vi "UI_Chose_Function.vi"() -> ()   [LabVIEW 2014]
panel:
  in  "报警门限及工作条件修改":bool
  in  "载荷谱修改":bool
  in  "齿轮箱独立调试":T1
  in  "陪试单元独立调试":T2
  in  "加载单元独立调试":T3
  in  "试验单元独立调试":T4
  in  "退出登录":T5
  in  "用户管理":T6
  in  "历史信息":T7
  in  "开始试验":T8
  # "轴承测试系统"
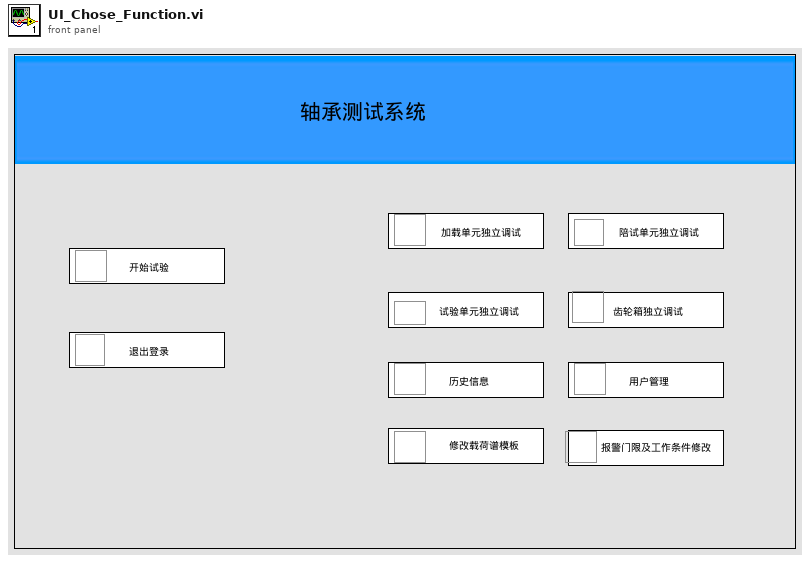
[diagram p1: front panel]
types:
  T1 = typedef "齿轮箱独立测试.ctl" = bool
  T2 = typedef "陪试单元独立调试.ctl" = bool
  T3 = typedef "加载单元独立调试.ctl" = bool
  T4 = typedef "试验单元独立调试.ctl" = bool
  T5 = typedef "退出登录1.ctl" = bool
  T6 = typedef "用户管理.ctl" = bool
  T7 = typedef "历史信息.ctl" = bool
  T8 = typedef "开始试验.ctl" = bool
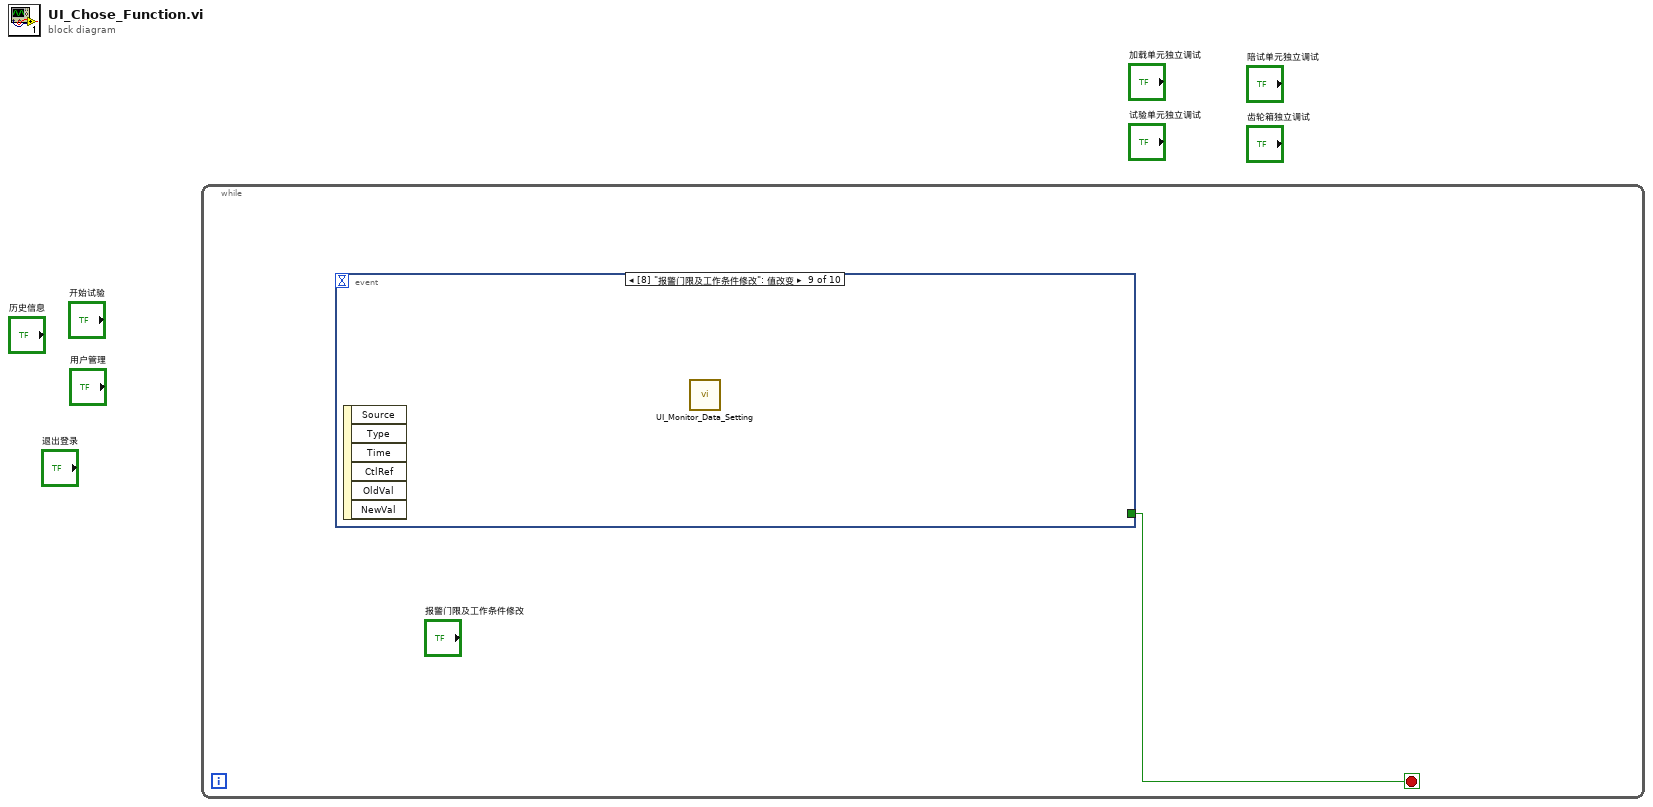
[diagram p0: block diagram]
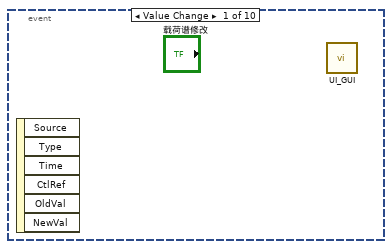
[diagram p2: hidden frame]
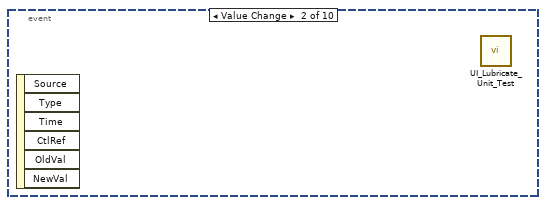
[diagram p3: hidden frame]
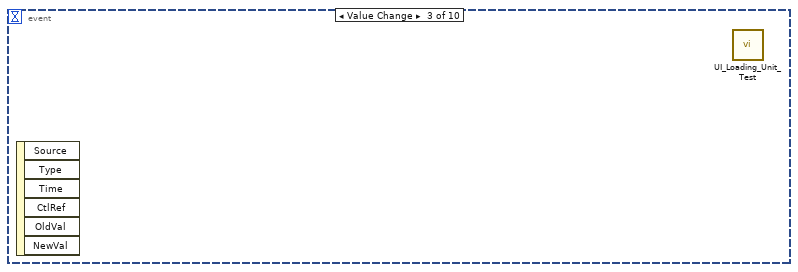
[diagram p4: hidden frame]
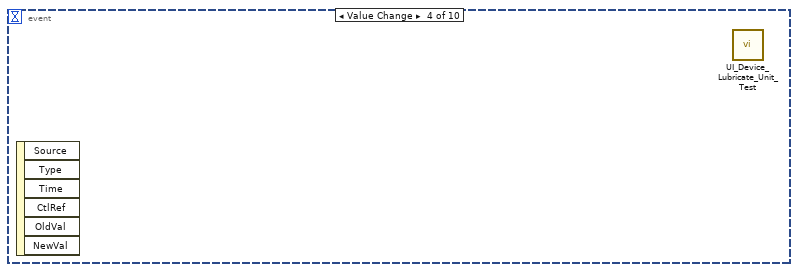
[diagram p5: hidden frame]
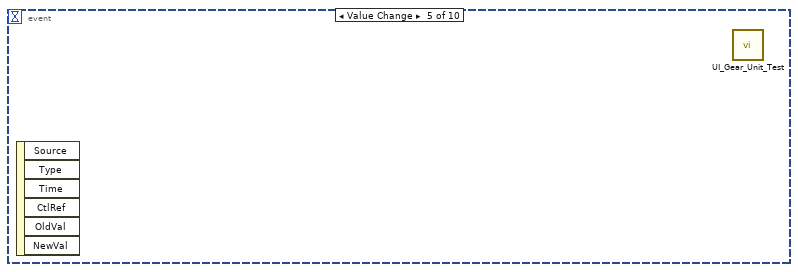
[diagram p6: hidden frame]
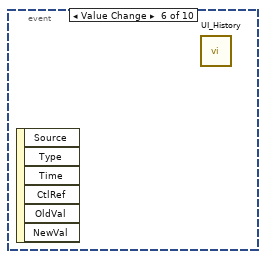
[diagram p7: hidden frame]
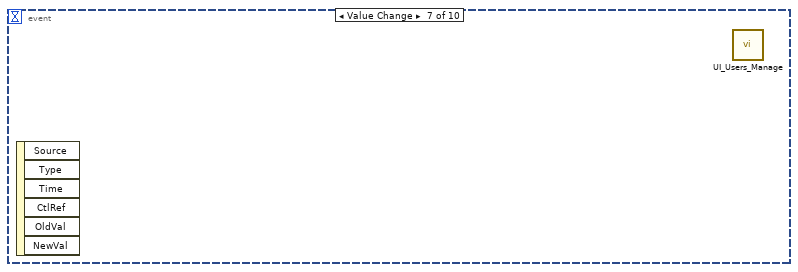
[diagram p8: hidden frame]
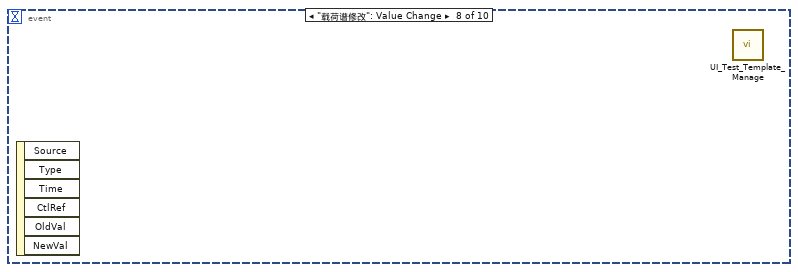
[diagram p9: hidden frame]
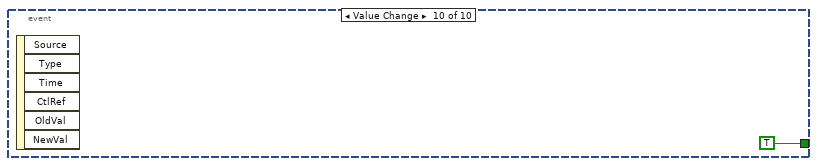
[diagram p10: hidden frame]
diagram:
  n1 = while {
    stop <- w1 stop-if-true
    n2 = event shown="[8] \"报警门限及工作条件修改\": 值改变" {
      selector: _ -> [_ _ _ _ _ _ _ _ _ _]
      dyn-events: _ -> [_ _ _ _ _ _ _ _ _ _]
      timeout: _ -> [_ _ _ _ _ _ _ _ _ _]
      tunnel: [_ _ _ _ _ _ _ _ _ TRUE] -> w1
      event Value Change {
        n3 = event-data() -> ()  [unwired: 1 in, 6 out]
        n4 = call "UI_GUI.vi"() -> ()  [unwired: 12 in]
      }
      event Value Change {
        n5 = event-data() -> ()  [unwired: 1 in, 6 out]
        n6 = call "UI_Lubricate_Unit_Test.vi"() -> ()  [unwired: 12 in]
      }
      event Value Change {
        n7 = event-data() -> ()  [unwired: 1 in, 6 out]
        n8 = call "UI_Loading_Unit_Test.vi"() -> ()  [unwired: 12 in]
      }
      event Value Change {
        n9 = event-data() -> ()  [unwired: 1 in, 6 out]
        n10 = call "UI_Device_Lubricate_Unit_Test.vi"() -> ()  [unwired: 12 in]
      }
      event Value Change {
        n11 = event-data() -> ()  [unwired: 1 in, 6 out]
        n12 = call "UI_Gear_Unit_Test.vi"() -> ()  [unwired: 12 in]
      }
      event Value Change {
        n13 = event-data() -> ()  [unwired: 1 in, 6 out]
        n14 = call "UI_History.vi"() -> ()  [unwired: 12 in]
      }
      event Value Change {
        n15 = event-data() -> ()  [unwired: 1 in, 6 out]
        n16 = call "UI_Users_Manage.vi"() -> ()  [unwired: 12 in]
      }
      event "载荷谱修改": Value Change {
        n17 = event-data() -> ()  [unwired: 1 in, 6 out]
        n18 = call "UI_Test_Template_Manage.vi"() -> ()  [unwired: 12 in]
      }
      event "报警门限及工作条件修改": Value Change {
        n19 = event-data() -> ()  [unwired: 1 in, 6 out]
        n20 = call "UI_Monitor_Data_Setting.vi"() -> ()  [unwired: 12 in]
      }
      event Value Change {
        n21 = event-data() -> ()  [unwired: 1 in, 6 out]
      }
    }
  }
